vi "IDS Fix ROI Size.vi"(0 "Requested Value":i32, 11 "Allowed Increment":i32) -> (8 "Resulting Value":i32)   [LabVIEW 2025]
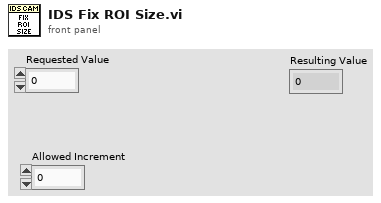
[diagram p1: front panel]
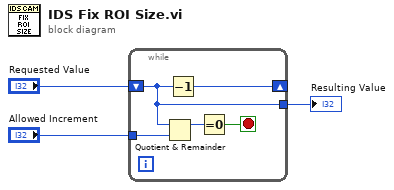
[diagram p0: block diagram]
diagram:
  n1 = while {
    shift-right: [w5] -> _
    shift-left: "Requested Value" -> [w4]
    tunnel: "Allowed Increment" -> [w8]
    tunnel: [w4] -> w1
    stop <- w6 stop-if-true
    n2 = Quotient & Remainder(x=w4, y=w8) -> (x-y*floor(x/y)=w7:i32)  [unwired: 1 out]
    n3 = Decrement(x=w4) -> (x-1=w5:i32)
    n4 = Equal To 0?(x=w7) -> (x = 0?=w6:bool)
  }
  "Resulting Value" <- w1
